vi "Keithley 2100 Series Read Single.vi"() -> ()   [LabVIEW 2020]
doc: "This example shows how to select a function and read a measurement."
uses:
  Public/Configure/Configure DC Volts.vi
  Public/Configure/Configure AC Volts.vi
  Public/Configure/Configure DC Current.vi
  Public/Configure/Configure AC Current.vi
  Public/Configure/Configure 2 Wire Resistance.vi
  Public/Configure/Configure 4 Wire Resistance.vi
  Keithley 2100 Series.lvlib
panel:
  out "Measurement":dbl
  in  "Measure":bool
  in  "Function (0: DC Volts)":u16(ring) items=["DC Volts", "AC Volts", "DC Current", "AC Current", "2-Wire Resistance", "4-Wire Resistance"]
  in  "VISA resource name":refnum<visa-resource-name>="GPIB::16"
  # "This example shows how to select a function, \nuse a bus trigger, and read a measurement.\n\nInstructions:\n1. Select a function.\n2. Run the VI\n3. Press the \"Measure\" button to take a measurement."
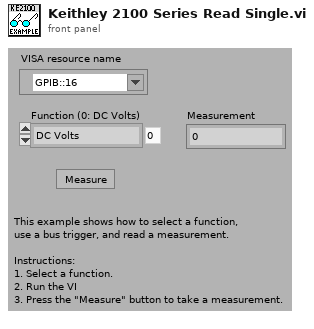
[diagram p1: front panel]
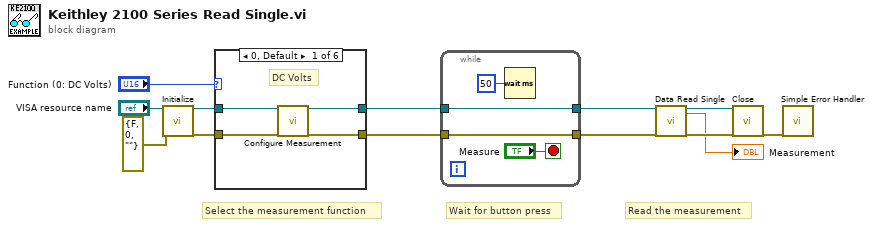
[diagram p0: block diagram]
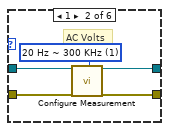
[diagram p2: hidden frame]
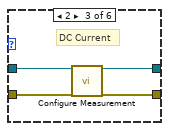
[diagram p3: hidden frame]
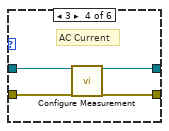
[diagram p4: hidden frame]
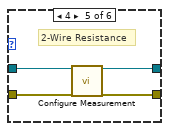
[diagram p5: hidden frame]
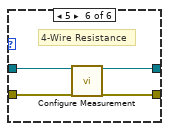
[diagram p6: hidden frame]
diagram:
  # "Read the measurement"
  # "Wait for button press"
  # "Select the measurement function"
  n1 = call "Initialize.vi"("VISA resource name"="VISA resource name", "error in (no error)"=errorcluster {"status"=FALSE, "code"=0, "source"=""}) -> ("VISA resource name out"=w10:refnum<visa-resource-name>, "error out"=w13:errorcluster)  [unwired: 16 in]
  n2 = case shown="0, Default" "Function (0: DC Volts)" {
    tunnel: w13 -> [w17 w22 w26 w30 w34 w38]
    tunnel: w10 -> [w16 w21 w25 w29 w33 w37]
    tunnel: [w15 w20 w24 w28 w32 w36] -> w3
    tunnel: [w14 w19 w23 w27 w31 w35] -> w4
    frame 0, Default {
      # "DC Volts"
      n3 = call-poly "Configure Measurement.vi"("VISA resource name"=w16, "error in (no error)"=w17) -> ("VISA resource name out"=w14:refnum<visa-resource-name>, "error out"=w15:errorcluster)  [unwired: 16 in]
    }
    frame 1 {
      w18 = u16 1 items=["3 Hz ~ 300 KHz", "20 Hz ~ 300 KHz", "200 Hz ~ 300 KHz"] ("Bandwidth (20 Hz)")
      # "AC Volts"
      n4 = call-poly "Configure Measurement.vi"("VISA resource name"=w21, "error in (no error)"=w22, "Bandwidth (20 Hz)"=w18) -> ("VISA resource name out"=w19:refnum<visa-resource-name>, "error out"=w20:errorcluster)  [unwired: 15 in]
    }
    frame 2 {
      # "DC Current"
      n5 = call-poly "Configure Measurement.vi"("VISA resource name"=w25, "error in (no error)"=w26) -> ("VISA resource name out"=w23:refnum<visa-resource-name>, "error out"=w24:errorcluster)  [unwired: 16 in]
    }
    frame 3 {
      # "AC Current"
      n6 = call-poly "Configure Measurement.vi"("VISA resource name"=w29, "error in (no error)"=w30) -> ("VISA resource name out"=w27:refnum<visa-resource-name>, "error out"=w28:errorcluster)  [unwired: 16 in]
    }
    frame 4 {
      # "2-Wire Resistance"
      n7 = call-poly "Configure Measurement.vi"("VISA resource name"=w33, "error in (no error)"=w34) -> ("VISA resource name out"=w31:refnum<visa-resource-name>, "error out"=w32:errorcluster)  [unwired: 16 in]
    }
    frame 5 {
      # "4-Wire Resistance"
      n8 = call-poly "Configure Measurement.vi"("VISA resource name"=w37, "error in (no error)"=w38) -> ("VISA resource name out"=w35:refnum<visa-resource-name>, "error out"=w36:errorcluster)  [unwired: 16 in]
    }
  }
  n9 = while {
    tunnel: w4 -> [w42]
    tunnel: w3 -> [w41]
    tunnel: [w42] -> w2
    tunnel: [w41] -> w1
    stop <- "Measure" stop-if-true
    n10 = Wait (ms)(milliseconds to wait=u32 50) -> ()  [unwired: 1 out]
  }
  n11 = call "Data Read Single.vi"("VISA resource name"=w2, "error in (no error)"=w1) -> ("VISA resource name out"=w11:refnum<visa-resource-name>, "Measurement"=→"Measurement":dbl, "error out"=w12:errorcluster)  [unwired: 15 in]
  n12 = call "Close.vi"("VISA resource name"=w11, "error in (no error)"=w12) -> ("error out"=w9:errorcluster)  [unwired: 17 in]
  n13 = call <vilib>:"Simple Error Handler.vi"("error in (no error)"=w9) -> ()  [unwired: 4 in, 5 out]
